vi "main.vi"() -> ()   [LabVIEW 2011]
uses:
  <vilib>/picture/picture.llb/Draw True-Color Pixmap.vi
panel:
  out "Voltage":dbl(graph)
  in  "Path for log file":path
  out "Tank  2":dbl(graph)
  out "Tank 1":dbl(graph)
  out "Apparatus F":T1 {"volt1" format="%.2f"; "A.2" format="%.2f"; "Tank 2" scale=0.0..20.0; "A.1" format="%.2f"; "Tank 1" scale=0.0..20.0}
  out "Packet Received":string
  in  "Read 2":i32=9002
  out "KTH  Automatic Control \nWicompi Project":picture
  in  "enabled":bool
  # "Network Cooridinated Serial Port"
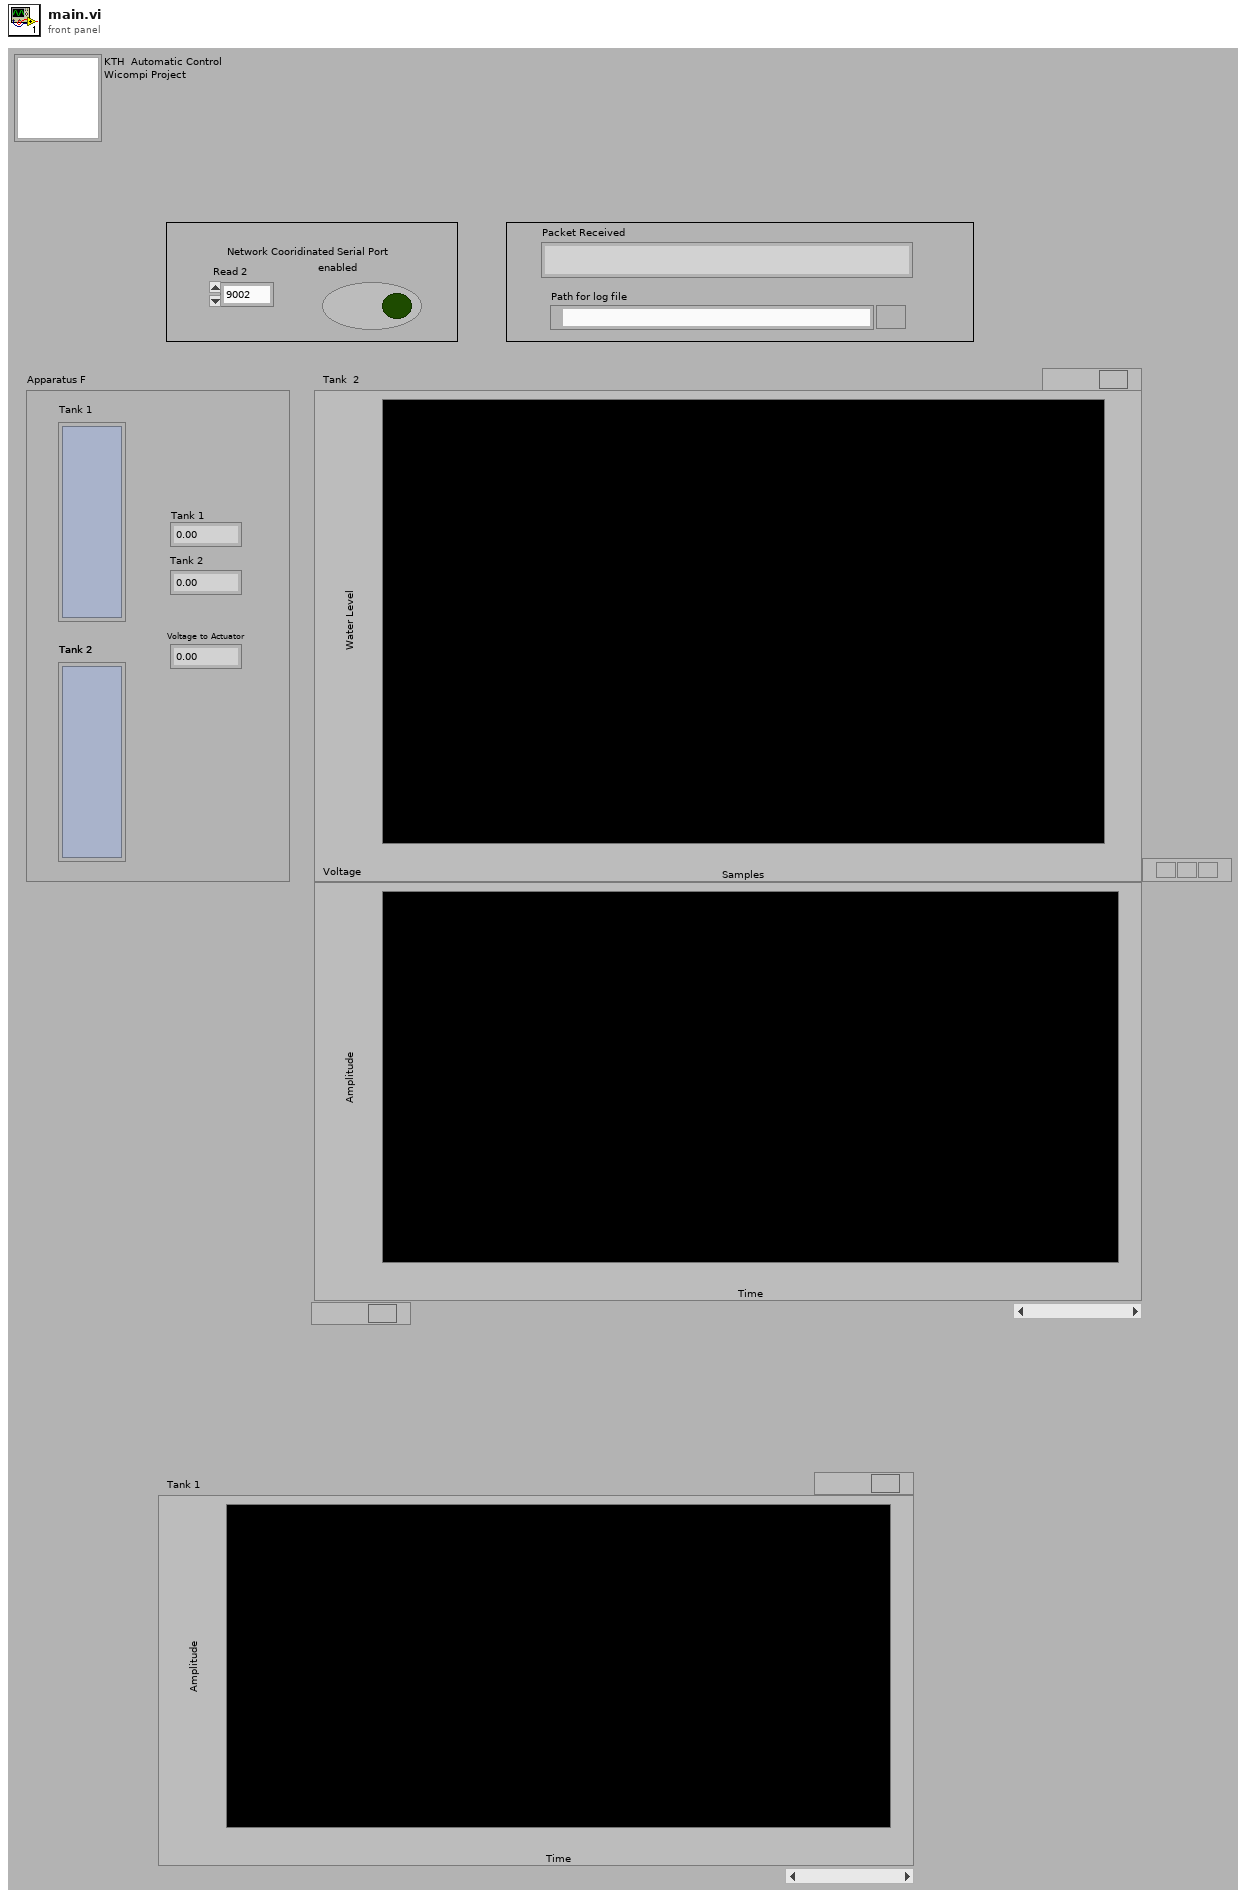
[diagram p1: front panel]
types:
  T1 = cluster{"Tank 1":dbl, dbl, "Tank 2":dbl, dbl, dbl}
  T2 = enum16{"open", "replace", "create", "open or create", "replace or create", "replace or create with confirmation"}
  T3 = typedef "imagedata.ctl" = cluster{"image type":i32, "image depth":i32, "image":u8[], "mask":u8[], "colors":u32[], "Rectangle":cluster{"left":i16, "top":i16, "right":i16, "bottom":i16}}
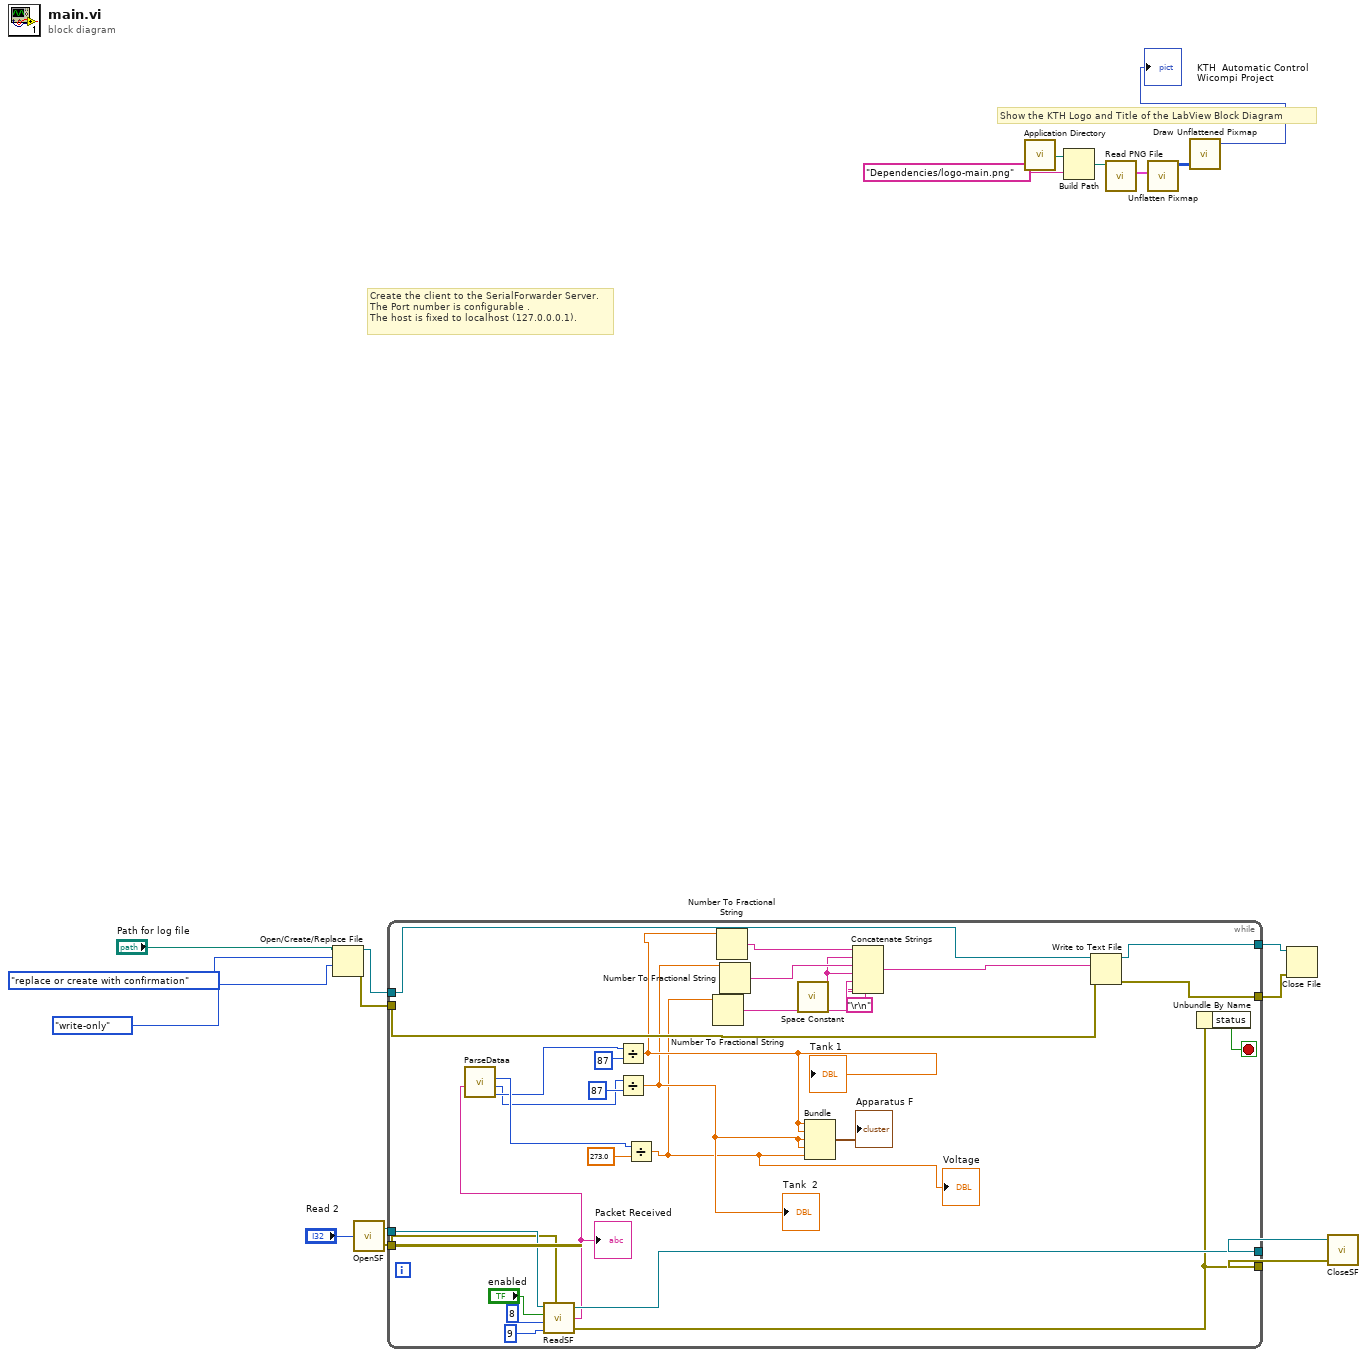
[diagram p0: block diagram]
diagram:
  # "Create the client to the SerialForwarder Server.\nThe Port number is configurable . \nThe host is fixed to localhost (127.0.0.0.1)."
  # "Show the KTH Logo and Title of the LabView Block Diagram"
  n1 = Open/Create/Replace File(file path (use dialog)="Path for log file", operation (0:open)=T2."replace or create with confirmation", access (0:read/write)=enum16{"read/write", "read-only", "write-only"}."write-only") -> (refnum out=w5:refnum<file>, error out=w4:errorcluster)  [unwired: 3 in, 1 out]
  n2 = call "OpenSF.vi"("Port Number"="Read 2") -> ("error out"=w11:errorcluster, "connection ID"=w10:refnum<k5>)
  n3 = while {
    tunnel: w10 -> [w42]
    tunnel: w11 -> [w41]
    tunnel: [w32] -> w9
    tunnel: [w43] -> w8
    tunnel: [w29] -> w7
    tunnel: [w28] -> w6
    tunnel: w5 -> [w27]
    tunnel: w4 -> [w26]
    stop <- w47 stop-if-true
    n4 = call "ReadSF.vi"("connection ID in"=w42, "error in"=w41, "enabled"="enabled", "bytes to read"=8, "header size"=9) -> ("connection ID out"=w43:refnum<k5>, "string"=w40:string, "error out"=w32:errorcluster)  [unwired: 1 in]
    "Packet Received" <- w40
    n5 = call "ParseDataa.vi"("data out"=w40) -> ("Tank1"=w34:u16, "Tank2"=w33:u16, "Voltage"=w35:u16)  [unwired: 7 in, 1 out]
    n6 = Divide(x=w34, y=u16 87) -> (x/y=w25:dbl)
    "Tank 1" <- w25
    n7 = Divide(x=w33, y=u16 87) -> (x/y=w24:dbl)
    "Tank  2" <- w24
    n8 = Divide(x=w35, y=273.0) -> (x/y=w19:dbl)
    "Voltage" <- w19
    n9 = Number To Fractional String(number=w19) -> (F-format string=w22:string)  [unwired: 3 in]
    n10 = Number To Fractional String(number=w25) -> (F-format string=w30:string)  [unwired: 3 in]
    n11 = Number To Fractional String(number=w24) -> (F-format string=w23:string)  [unwired: 3 in]
    n12 = call <vilib>:"Space Constant.vi"() -> ("String"=w21:string)
    n13 = Bundle(w25, w25, w24, w24, w19) -> (→"Apparatus F":cluster{dbl, dbl, dbl, dbl, dbl})  [unwired: 1 in]
    n14 = Concatenate Strings(w30, w21, w23, w21, w22, "\r\n") -> (w31:string)
    n15 = Write to Text File(file (use dialog)=w27, text=w31, error in=w26) -> (refnum out=w29:refnum<file>, error out=w28:errorcluster)  [unwired: 1 in, 1 out]
    n16 = Unbundle By Name(w32) -> ("status"=w47:bool)
  }
  n17 = call <vilib>:"Application Directory.vi"() -> ("Application Directory"=w15:path)
  n18 = Build Path(base path=w15, name or relative path="Dependencies/logo-main.png") -> (appended path=w16:path)
  n19 = call <vilib>:"Read PNG File.vi"("path to PNG file"=w16) -> ("image data"=w18:T3)  [unwired: 8 in, 2 out]
  n20 = call <vilib>:"Unflatten Pixmap.vi"("image data"=w18) -> ("24-bit pixmap"=w17:u32[][])  [unwired: 4 in, 6 out]
  n21 = call-poly <vilib>:"Draw Unflattened Pixmap.vi"("data (RGB format)"=w17) -> ("new picture"=→"KTH  Automatic Control \nWicompi Project":picture)  [unwired: 8 in]
  n22 = Close File(refnum=w7, error in=w6) -> ()  [unwired: 2 out]
  n23 = call "CloseSF.vi"("error out"=w9, "connection ID"=w8) -> ()  [unwired: 1 in]
